vi "ReleaseFrame.vi"(6 "frameHandle":i64, 8 "pData":u8[](array[numeric]), 9 "pLbFrame":T1, 10 "handle":i64, 11 "error in (no error)":errorcluster) -> (3 "error out":errorcluster)   [LabVIEW 2016]
uses:
  MVSDKmd.dll
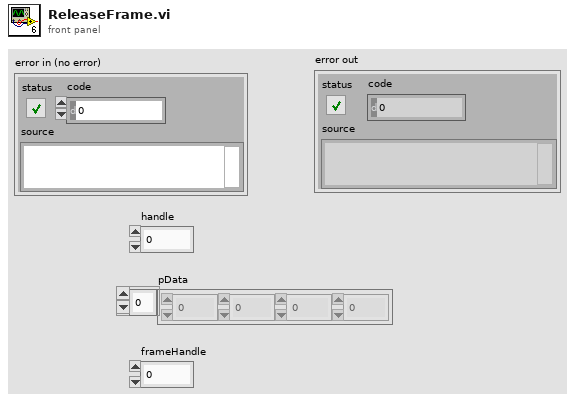
[diagram p1: front panel]
types:
  T1 = cluster{"blockId":u64, "status":u32, "width":u32, "height":u32, "size":u32, "pixelFormat":u32, "timeStamp":u64, "chunkCount":u32, "paddingX":u32, "paddingY":u32, "recvFrameTime":u32}
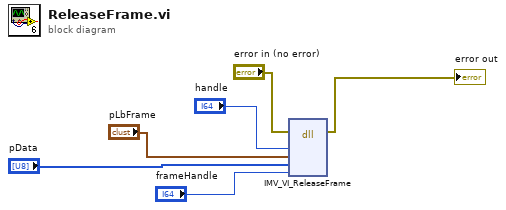
[diagram p0: block diagram]
diagram:
  n1 = dll-call lib="MVSDKmd.dll" fn="IMV_VI_ReleaseFrame"(error in="error in (no error)", "handle"="handle", "pFrame"="pLbFrame", "pData"="pData", "frameHandle"="frameHandle") -> (error out=→"error out":errorcluster)  [unwired: 7 in, 1 out]
